vi "Decode Message Data (Test End).vi"(7 "Message Data":variant, 11 "error in":errorcluster) -> (4 "Test":T1, 8 "Error":errorcluster, 15 "error out":errorcluster)   [LabVIEW 2016, in "Hall Effect Library.lvlib"]
uses:
  Hall Effect Library.lvlib
  Controls/Tests.ctl
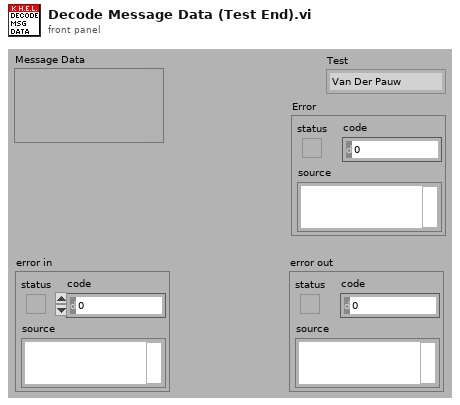
[diagram p1: front panel]
types:
  T1 = typedef "Hall Effect Library.lvlib/Tests.ctl" = enum16{"Van Der Pauw", "Hall Effect", "Bar Sample Resistivity", "Bar Sample Hall ", "6-Contact Sample Resistivity", "6-Contact Sample Hall", "8-Contact Sample Resistivity", "8-Contact Sample Hall", ""}
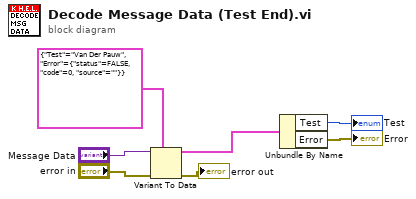
[diagram p0: block diagram]
diagram:
  n1 = Variant To Data(error in="error in", type=cluster{"Test":T1, "Error":errorcluster} {"Test"=enum."Van Der Pauw", "Error"={"status"=FALSE, "code"=0, "source"=""}}, Variant="Message Data") -> (data=w3:cluster{"Test":T1, "Error":errorcluster}, error out=→"error out":errorcluster)
  n2 = Unbundle By Name(w3) -> ("Test"=→"Test":T1, "Error"=→"Error":errorcluster)
